vi "HeartSoundIndices.vi"(11 "RR intervals [ms]":dbl[](array[numeric])) -> (0 "pNN50 [%]":dbl format="%0.2f", 1 "rMSSD  [ms]":dbl format="%0.2f", 2 "sdRR [ms]":dbl format="%0.2f", 3 "Mean RR [ms]":dbl format="%0.2f", 5 "Mean heart rate [BPM]":dbl)   [LabVIEW 2014, in "Phonocardiography.lvlib"]
uses:
  Phonocardiography.lvlib
  <vilib>/Analysis/NI_AALBase.lvlib
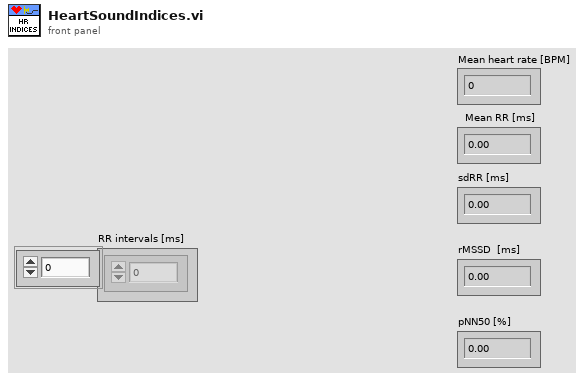
[diagram p1: front panel]
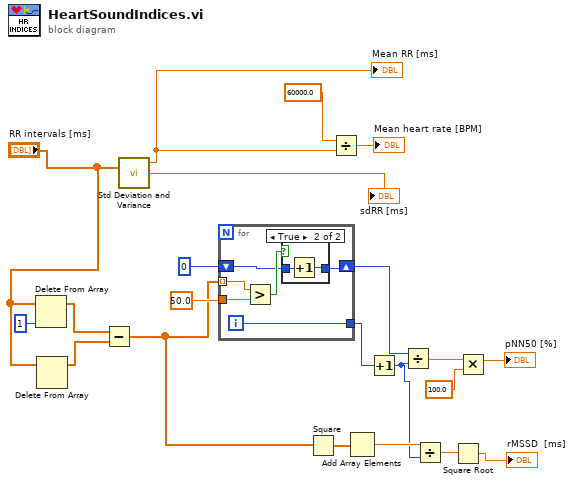
[diagram p0: block diagram]
diagram:
  n1 = Delete From Array(array="RR intervals [ms]", index=1) -> (array with subset deleted=w16:dbl[])  [unwired: 1 in, 1 out]
  n2 = Delete From Array(array="RR intervals [ms]") -> (array with subset deleted=w15:dbl[])  [unwired: 2 in, 1 out]
  n3 = Subtract(x=w16, y=w15) -> (x-y=w7:dbl[])
  n4 = call <vilib>:"Std Deviation and Variance.vi"("X"="RR intervals [ms]") -> ("mean"=w20:dbl, "standard deviation"=→"sdRR [ms]":dbl)  [unwired: 1 in, 1 out]
  "Mean RR [ms]" <- w20
  n5 = for {
    tunnel: 50.0 ("y") -> [w26]
    tunnel: w7 -> [w27] mode=indexing
    shift-right: [w23] -> w9
    shift-left: 0 ("index") -> [w24]
    tunnel: [w22] -> w8
    i -> [w22]
    n6 = Greater?(x=w27, y=w26) -> (0:w25:bool)
    n7 = case shown="True" w25 {
      tunnel: w24 -> [w28 w30]
      tunnel: [w28 w29] -> w23
      frame False {
      }
      frame True {
        n8 = Increment(x=w30) -> (x+1=w29:i32)
      }
    }
  }
  n9 = Square(x=w7) -> (x^2=w6:dbl[])
  n10 = Divide(x=60000.0, y=w20) -> (x/y=→"Mean heart rate [BPM]":dbl)
  n11 = Add Array Elements(numeric array=w6) -> (sum=w5:dbl)
  n12 = Increment(x=w8) -> (x+1=w4:i32)
  n13 = Divide(x=w9, y=w4) -> (x/y=w14:dbl)
  n14 = Divide(x=w5, y=w4) -> (x/y=w3:dbl)
  n15 = Square Root(x=w3) -> (sqrt(x)=→"rMSSD  [ms]":dbl)
  n16 = Multiply(x=w14, y=100.0) -> (x*y=→"pNN50 [%]":dbl)
